vi "FTW-JSON-LexicalScan-String-Escaped.vi"(0 "JSON String":T1, 11 "error in":errorcluster) -> (4 "JSON String Out":T1, 8 "String":string, 14 "Found Match?":bool, 15 "error out":errorcluster)   [LabVIEW 2015]
uses:
  FTW-JSON-LexicalScan.ctl
panel:
  # "Inputs"
  # "Outputs"
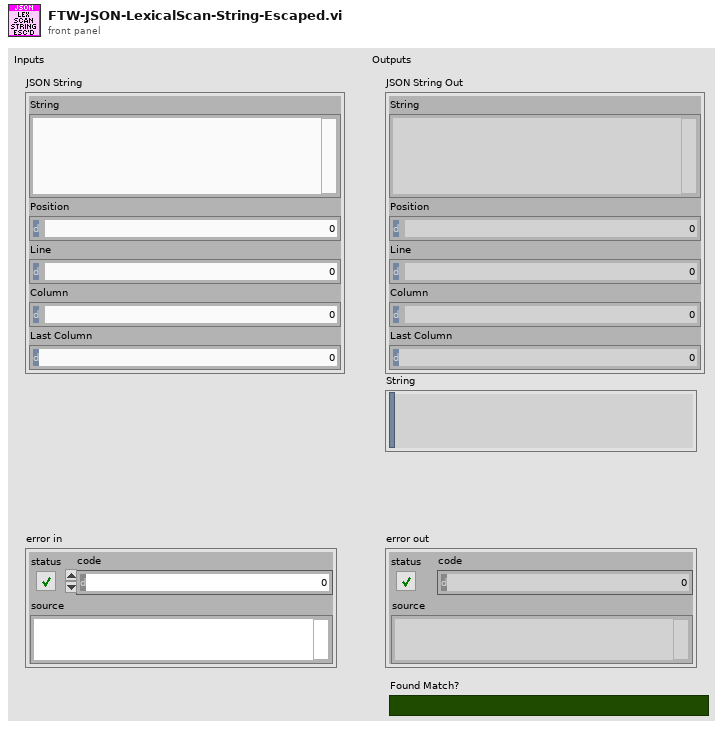
[diagram p1: front panel]
types:
  T1 = typedef "FTW-JSON-LexicalScan.ctl" = cluster{"String":string, "Position":i32, "Line":i32, "Column":i32, "Last Column":i32}
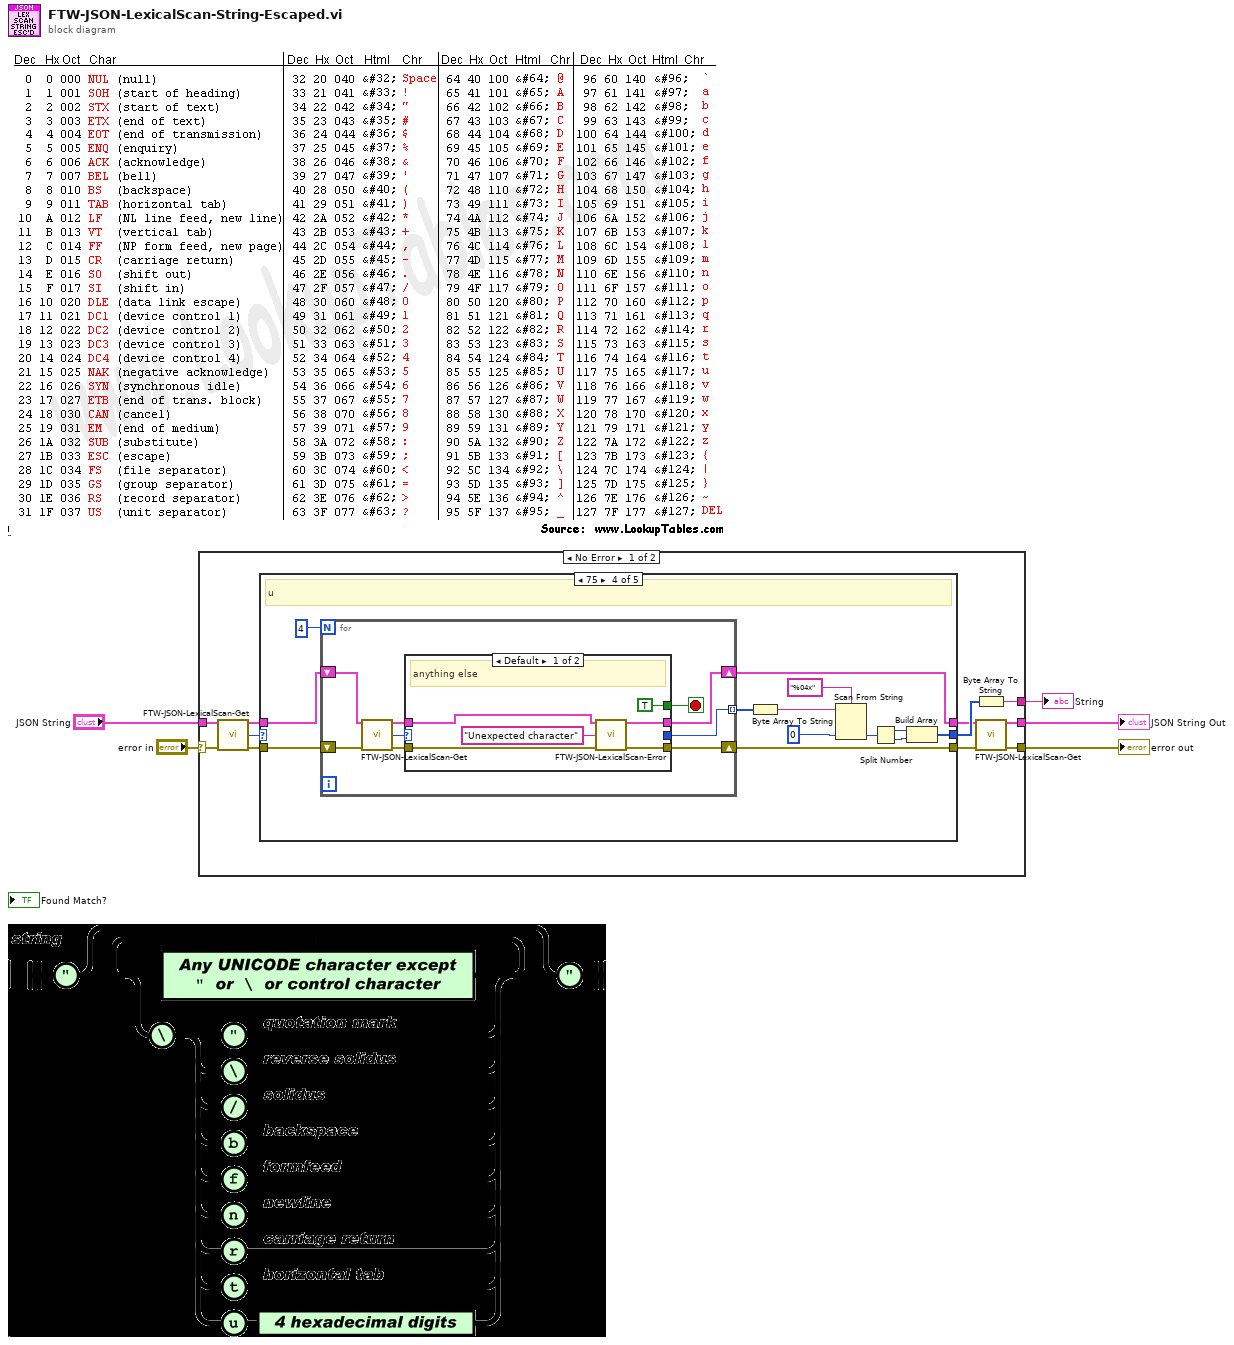
[diagram p0: block diagram]
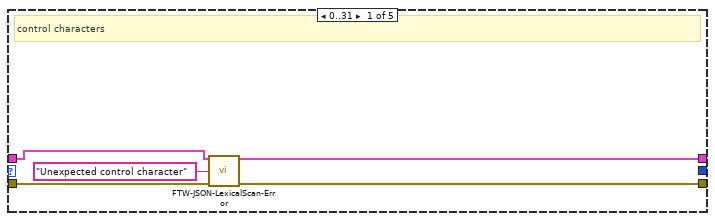
[diagram p2: hidden frame]
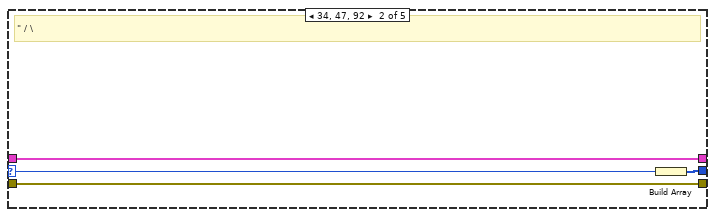
[diagram p3: hidden frame]
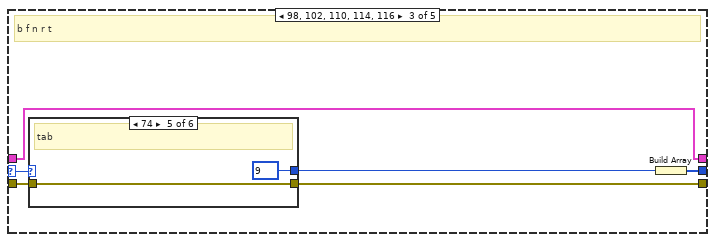
[diagram p4: hidden frame]
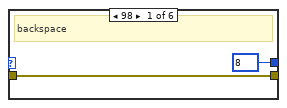
[diagram p5: hidden frame]
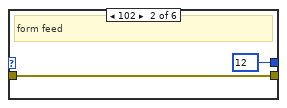
[diagram p6: hidden frame]
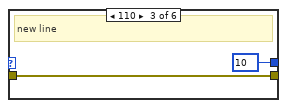
[diagram p7: hidden frame]
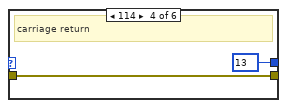
[diagram p8: hidden frame]
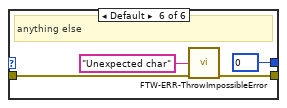
[diagram p9: hidden frame]
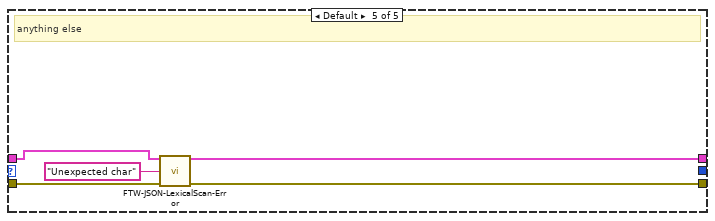
[diagram p11: hidden frame]
diagram:
  n1 = case shown="No Error" "error in" {
    selector: "error in" -> [w16 w82]
    tunnel: [w8 w82] -> w5
    tunnel: "JSON String" -> [w11 _]
    tunnel: [w6 _] -> w2
    tunnel: [w13 _] -> w4
    frame No Error {
      n2 = call "FTW-JSON-LexicalScan-Get.vi"("JSON String"=w11, "error in"=w16) -> ("JSON String Out"=w10:T1, "Char"=w9:u8, "error out"=w12:errorcluster)  [unwired: 11 in]
      n3 = case shown="75" w9 {
        selector: w9 -> [_ w24 w27 _ _]
        tunnel: w12 -> [w21 w25 w29 w58 w81]
        tunnel: [w20 w25 w28 w55 w80] -> w15
        tunnel: [_ w23 w30 w46 _] -> w14
        tunnel: w10 -> [w19 w22 w31 w57 w79]
        tunnel: [w18 w22 w31 w56 w78] -> w7
        frame 0..31 {
          # "control characters"
          n4 = call "FTW-JSON-LexicalScan-Error.vi"("JSON String"=w19, "Error String"="Unexpected control character" ("Error Message"), "error in"=w21) -> ("JSON String Out"=w18:T1, "error out"=w20:errorcluster)  [unwired: 11 in]
        }
        frame 34, 47, 92 {
          # "\" / \\"
          n5 = Build Array(w24) -> (w23:u8[])
        }
        frame 98, 102, 110, 114, 116 {
          # "b f n r t"
          n6 = case shown="74" w27 {
            tunnel: w29 -> [w33 w35 w37 w39 w41 w45]
            tunnel: [w33 w35 w37 w39 w41 w44] -> w28
            tunnel: [u8 8 u8 12 u8 10 u8 13 u8 9 u8 0] -> w26
            frame 98 {
              # "backspace"
            }
            frame 102 {
              # "form feed"
            }
            frame 110 {
              # "new line"
            }
            frame 114 {
              # "carriage return"
            }
            frame 116 {
              # "tab"
            }
            frame Default {
              # "anything else"
              n7 = call "FTW-ERR-ThrowImpossibleError.vi"("Reason this error should never happen"="Unexpected char" ("Error Message"), "error in"=w45) -> ("error out"=w44:errorcluster)  [unwired: 13 in]
            }
          }
          n8 = Build Array(w26) -> (w30:u8[])
        }
        frame 117 {
          # "u"
          n9 = for {
            N: 4 -> [_]
            shift-right: [w66] -> w55
            shift-left: w58 -> [w67]
            shift-right: [w65] -> w56
            shift-left: w57 -> [w61]
            tunnel: [w63] -> w53 mode=indexing
            stop <- w64 stop-if-true
            n10 = call "FTW-JSON-LexicalScan-Get.vi"("JSON String"=w61, "error in"=w67) -> ("JSON String Out"=w60:T1, "Char"=w59:u8, "error out"=w62:errorcluster)  [unwired: 11 in]
            n11 = case shown="Default" w59 {
              selector: w59 -> [_ w74]
              tunnel: w62 -> [w73 w76]
              tunnel: [w71 w76] -> w66
              tunnel: w60 -> [w70 w75]
              tunnel: [w69 w75] -> w65
              tunnel: [TRUE _] -> w64
              tunnel: [_ w74] -> w63
              frame Default {
                # "anything else"
                n12 = call "FTW-JSON-LexicalScan-Error.vi"("JSON String"=w70, "Error String"="Unexpected character" ("Error Message"), "error in"=w73) -> ("JSON String Out"=w69:T1, "error out"=w71:errorcluster)  [unwired: 11 in]
              }
              frame 48..57, 65..70 {
                # "hex chars"
              }
            }
          }
          n13 = Byte Array To String(unsigned byte array=w53) -> (string=w52:string)
          n14 = Scan From String(format string="%04x", input string=w52, default 1=u16 0 ("default value 1")) -> (output 1=w49:u16)  [unwired: 2 in, 3 out]
          n15 = Split Number(x=w49) -> (hi(x)=w48:u8, lo(x)=w47:u8)
          n16 = Build Array(w48, w47) -> (w46:u8[])
        }
        frame Default {
          # "anything else"
          n17 = call "FTW-JSON-LexicalScan-Error.vi"("JSON String"=w79, "Error String"="Unexpected char" ("Error Message"), "error in"=w81) -> ("JSON String Out"=w78:T1, "error out"=w80:errorcluster)  [unwired: 11 in]
        }
      }
      n18 = Byte Array To String(unsigned byte array=w14) -> (string=w13:string)
      n19 = call "FTW-JSON-LexicalScan-Get.vi"("JSON String"=w7, "error in"=w15) -> ("JSON String Out"=w6:T1, "error out"=w8:errorcluster)  [unwired: 11 in, 1 out]
    }
    frame Error {
    }
  }
  "String" <- w4
  "error out" <- w5
  "JSON String Out" <- w2
